vi "test_MonoGetConfig.vi"(6 "Delay between send and receive [ms]":i32=100, 7 "Test should pass":bool=TRUE, 8 "error in":errorcluster, 9 "tear down connection":bool=TRUE, 10 "set-up a connection":bool=TRUE, 11 "device selection":enum16{"monochromator", "CCD", "SCD"}(ring)) -> (0 "error out":errorcluster)   [LabVIEW 2023]
uses:
  Classes/Mono/configuration.ctl
  Classes/Mono/filterWheel.ctl
  Classes/Mono/grating.ctl
  Classes/Mono/mirror.ctl
  Classes/Mono/port.ctl
  Classes/Mono/Monochromator.lvclass
  C:/Projects/Horiba/horiba-labview-sdk/Source/Classes/GenericDevice/GenericDevice.lvclass
  <vilib>/addons/_JKI Toolkits/Caraya/classes/Assert/Assert Equal Value_Variant.vi
  <vilib>/addons/_JKI Toolkits/Caraya/classes/Assert/Assert Not Error.vi
  <vilib>/addons/_JKI Toolkits/Caraya/classes/Test/Test.lvclass
  <vilib>/addons/_JKI Toolkits/Caraya/classes/Assert/Assert.lvclass
  <vilib>/Hampel Software Engineering/HSE Logger/hse-logger.lvlib
panel:
  out "log-file path":path
  out "config-text pairs":string[][](array[string])=[["$.configuration.filterWheels", ""], ["$.configuration.gratings", "- blaze: 0\r  grooveDensity: 1800\r  positionIndex: 0\n- blaze: 0\r  grooveDensity: 1200\r  positionIndex: 1\n- blaze: 0\r  grooveDensity: 300\r  positionIndex: 2"], ["$.configuration.mirrors", "- location: 1\n- location: 2"], ["$.configuration.monoModel", "iHR320"], ["$.configuration.ports", "- monoPortLocation: 1\r  slitType: 2\n- monoPortLocation: 2\r  slitType: 2\n- monoPortLocation: 4\r  slitType: 2"], ["$.configuration.procuctId", "257"], ["$.configuration.serialNumber", ""]]
  out "config-JSON pairs":string[][](array[string])=[["$.configuration.filterWheels", "[]"], ["$.configuration.gratings", "[{\"blaze\":0,\"grooveDensity\":1800,\"positionIndex\":0},{\"blaze\":0,\"grooveDensity\":1200,\"positionIndex\":1},{\"blaze\":0,\"grooveDensity\":300,\"positionIndex\":2}]"], ["$.configuration.mirrors", "[{\"location\":1},{\"location\":2}]"], ["$.configuration.monoModel", "\"iHR320\""], ["$.configuration.ports", "[{\"monoPortLocation\":1,\"slitType\":2},{\"monoPortLocation\":2,\"slitType\":2},{\"monoPortLocation\":4,\"slitType\":2}]"], ["$.configuration.procuctId", "\"257\""], ["$.configuration.serialNumber", "\"\""]]
  out "config-JSON string":string="{\"configuration\":{\"CenterWavelength\":0,\"ChipHSpacing\":\"260\",\"ChipHeight\":\"256\",\"ChipName\":\"CCD30-11-1-275\",\"ChipSerialNumber\":\"20091-22-21\",\"ChipVSpacing\":\"260\",\"ChipWidth\":\"1024\",\"DeviceType\":\"HORIBA Scientific Syncerity\",\"FitParameters\":[0,1,0,0,0],\"Gains\":[{\"Info\":\"Best Dynamic Range\",\"Token\":1},{\"Info\":\"High Light\",\"Token\":0},{\"Info\":\"High Sensitivity\",\"Token\":2}],\"HardwareAvgAvailable\":\"False\",\"LineScan\":\"False\",\"ProductId\":\"13\",\"SerialNumber\":\"Camera SN:  2244\",\"Signals\":[{\"Events\":[{\"Name\":\"Ready For Trigger\",\"Token\":1,\"Types\":[{\"Name\":\"TTL Active Low\",\"Token\":1},{\"Name\":\"TTL Active High\",\"Token\":0}]},{\"Name\":\"Shutter Open\",\"Token\":3,\"Types\":[{\"Name\":\"TTL Active Low\",\"Token\":1},{\"Name\":\"TTL Active High\",\"Token\":0}]},{\"Name\":\"Start Experiment\",\"Token\":0,\"Types\":[{\"Name\":\"TTL Active Low\",\"Token\":1},{\"Name\":\"TTL Active High\",\"Token\":0}]},{\"Name\":\"Reserved-DO NOT USE\",\"Token\":2,\"Types\":[{\"Name\":\"TTL Active Low\",\"Token\":1},{\"Name\":\"TTL Active High\",\"Token\":0}]}],\"Name\":\"Signal Output\",\"Token\":0}],\"Speeds\":[{\"Info\":\" 1 MHz       \",\"Token\":1},{\"Info\":\"45 kHz       \",\"Token\":0},{\"Info\":\"500 kHz Wrap\",\"Token\":127},{\"Info\":\" 1 MHz Ultra \",\"Token\":2}],\"SupportedFeatures\":{\"CF_3PositionSlit\":\"False\",\"CF_CMOSOffsetCorrection\":\"False\",\"CF_Cleaning\":\"True\",\"CF_DSP\":\"False\",\"CF_DSPBin2X\":\"False\",\"CF_DelayAfterTrigger\":\"False\",\"CF_Delays\":\"False\",\"CF_EMCCD\":\"False\",\"CF_EShutter\":\"False\",\"CF_HDR\":\"False\",\"CF_Image\":\"True\",\"CF_MemorySlots\":\"True\",\"CF_Metadata\":\"False\",\"CF_MultipleExposeTimes\":\"False\",\"CF_MultipleSensors\":\"False\",\"CF_PulseSummation\":\"False\",\"CF_ROIs\":\"True\",\"CF_Signals\":\"True\",\"CF_Spectra\":\"True\",\"CF_TriggerQualifier\":\"False\",\"CF_Triggers\":\"True\"},\"Triggers\":[{\"Events\":[{\"Name\":\"Each - For Each Acq\",\"Token\":1,\"Types\":[{\"Name\":\"TTL Rising  Edge\",\"Token\":1},{\"Name\":\"TTL Falling Edge\",\"Token\":0}]},{\"Name\":\"Once - Start All\",\"Token\":0,\"Types\":[{\"Name\":\"TTL Rising  Edge\",\"Token\":1},{\"Name\":\"TTL Falling Edge\",\"Token\":0}]}],\"Name\":\"Trigger Input\",\"Token\":0}],\"Version\":\"Syncerity Ver 1.001.7.1\"}}"
  # "Connector Pane"
  # "Locals"
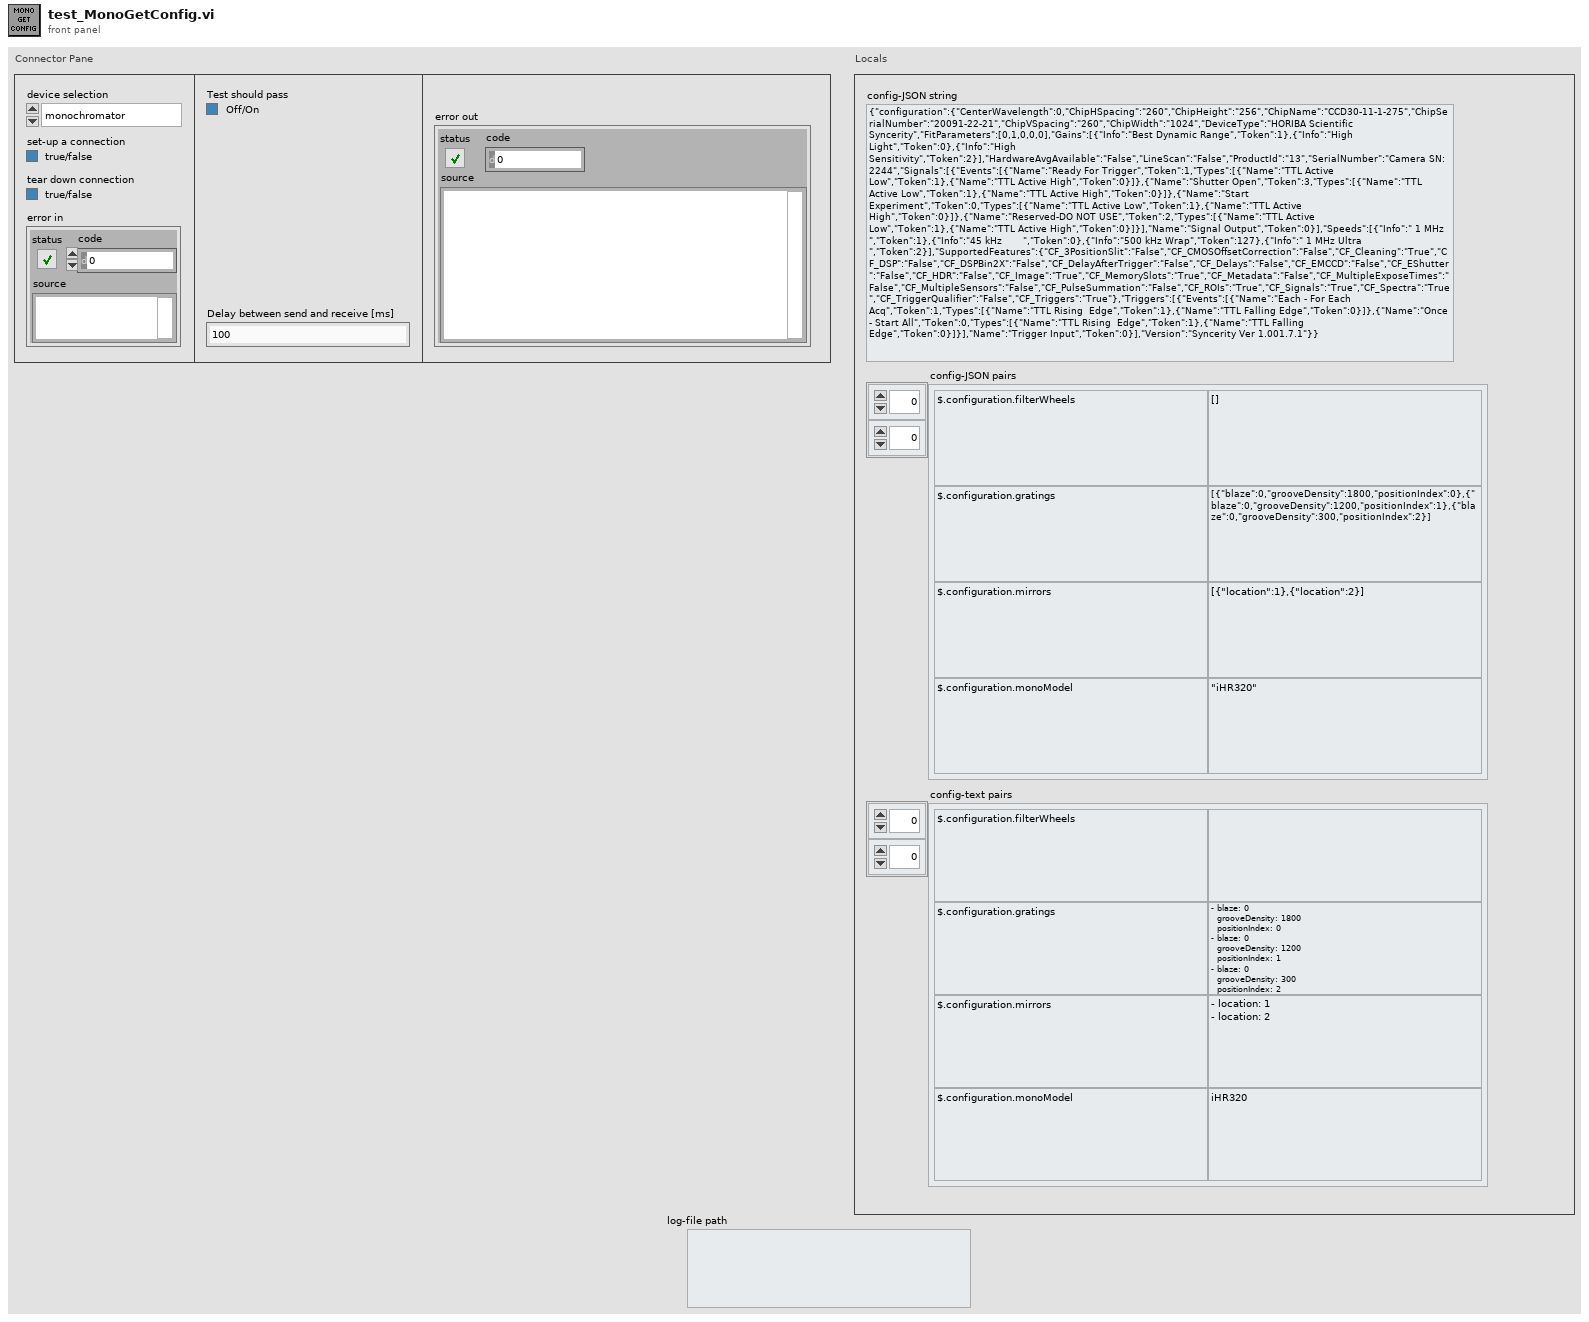
[diagram p1: front panel]
types:
  T1 = typedef "Monochromator.lvclass/configuration.ctl" = cluster{"filterWheels":T2[], "gratings":T3[], "mirrors":T4[], "model":string, "ports":T5[], "productId":string, "serialNumber":string}
  T2 = typedef "Monochromator.lvclass/filterWheel.ctl" = cluster{"locationId":i32}
  T3 = typedef "Monochromator.lvclass/grating.ctl" = cluster{"blaze":i32, "grooveDensity":i32, "positionIndex":i32}
  T4 = typedef "Monochromator.lvclass/mirror.ctl" = cluster{"locationId":i32}
  T5 = typedef "Monochromator.lvclass/port.ctl" = cluster{"locationId":i32, "slitType":i32}
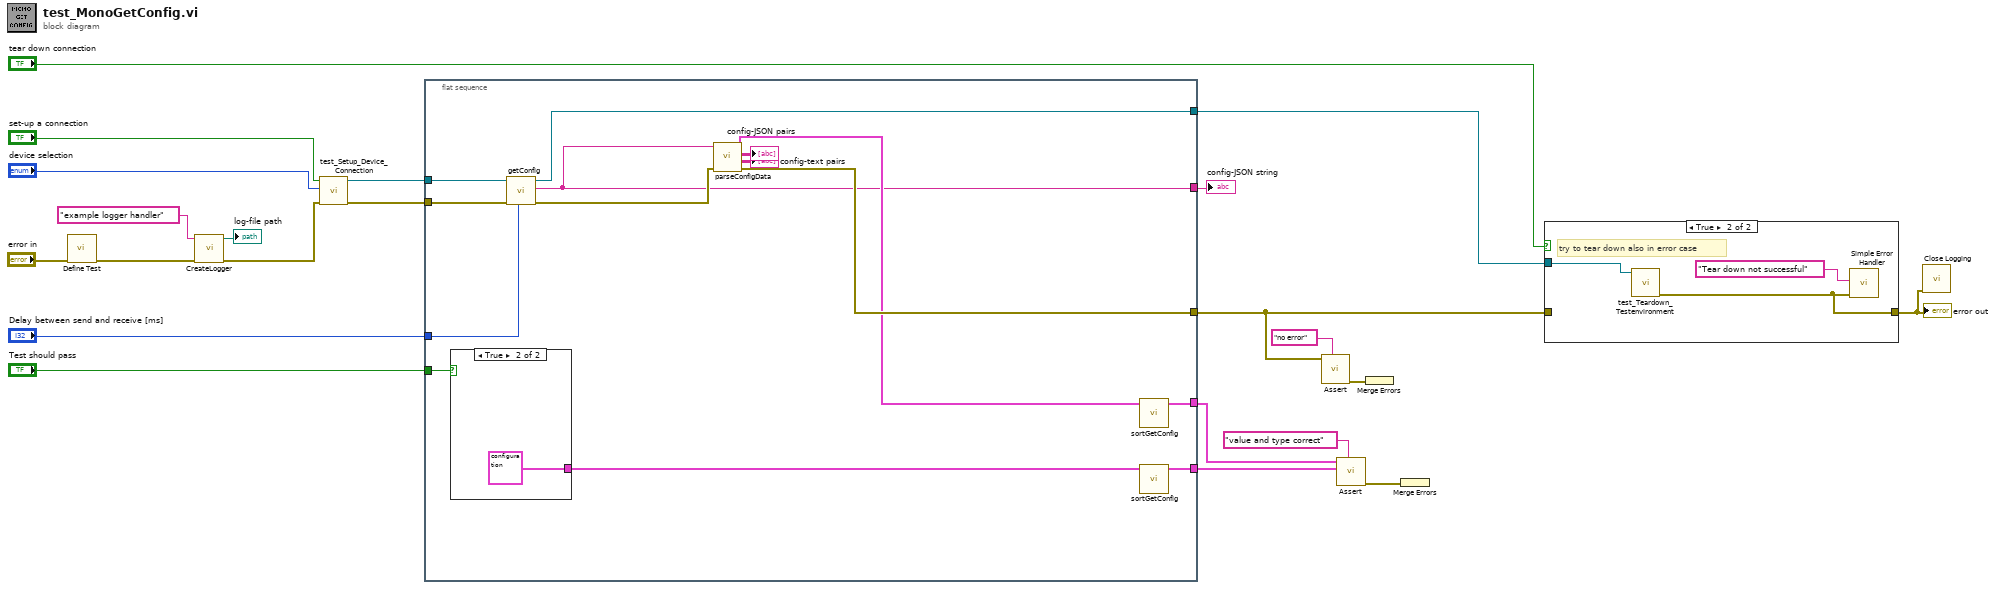
[diagram p0: block diagram]
diagram:
  n1 = call <vilib>:"Define Test.vi"("error in (no error)"="error in") -> ("error out"=w3:errorcluster)  [unwired: 9 in, 1 out]
  n2 = call "CreateLogger.vi"("error in (no error)"=w3, "Handler Name"="example logger handler") -> ("error out"=w2:errorcluster, "log-file path"=→"log-file path":path)  [unwired: 8 in]
  n3 = call "test_Setup_Device_Connection.vi"("error in (no error)"=w2, "device selection"="device selection", "set-up a connection"="set-up a connection") -> ("error out"=w10:errorcluster, "Monochromator.lvclass"=w7:refnum<class "Monochromator.lvclass">)  [unwired: 5 in, 2 out]
  n4 = flat-sequence {
    tunnel: [w26] -> w20
    tunnel: w10 -> [w36]
    tunnel: w7 -> [w35]
    tunnel: [w30] -> w14
    tunnel: "Test should pass" -> [w34]
    tunnel: [w33] -> w13
    tunnel: "Delay between send and receive [ms]" -> [w32]
    tunnel: [w23] -> w8
    tunnel: [w25] -> w6
    frame #0 {
      n5 = case shown="True" w34 {
        tunnel: [_ T1 {"filterWheels"=[], "gratings"=[{"blaze"=0, "grooveDensity"=1800, "positionIndex"=0}, {"blaze"=0, "grooveDensity"=1200, "positionIndex"=1}, {"blaze"=0, "grooveDensity"=300, "positionIndex"=2}], "mirrors"=[{"locationId"=1}, {"locationId"=2}], "model"="iHR320", "ports"=[{"locationId"=1, "slitType"=1}, {"locationId"=2, "slitType"=1}, {"locationId"=4, "slitType"=1}], "productId"="257", "serialNumber"=""} ("unsorted 2")] -> w24
        frame False {
        }
        frame True {
        }
      }
      n6 = call "getConfig.vi"("Delay between send and receive [ms]"=w32, "error in (no error)"=w36, "Monochromator in"=w35) -> ("error out"=w31:errorcluster, "config-JSON string"=w26:string, "Monochromator out"=w33:refnum<class "Monochromator.lvclass">)  [unwired: 6 in]
      n7 = call "parseConfigData.vi"("error in (no error)"=w31, "results-JSON string"=w26) -> ("error out"=w30:errorcluster, "config-text pairs"=→"config-text pairs":string[][], "config-JSON pairs"=→"config-JSON pairs":string[][], "config data"=w27:T1)  [unwired: 6 in]
      n8 = call "sortGetConfig.vi"("config data in"=w27) -> ("config data out"=w25:T1)  [unwired: 10 in]
      n9 = call "sortGetConfig.vi"("config data in"=w24) -> ("config data out"=w23:T1)  [unwired: 10 in]
    }
  }
  n10 = call-poly <vilib>:"Assert.vi"("Label"="no error" ("Label (VI Title)"), "Not Error?"=w14) -> ("error out"=w16:errorcluster)  [unwired: 8 in, 1 out]
  n11 = call-poly <vilib>:"Assert.vi"("Label"="value and type correct" ("Label (VI Title)"), "Y"=w8, "X"=w6) -> ("error out"=w21:errorcluster)  [unwired: 7 in, 1 out]
  n12 = Merge Errors(w16) -> ()  [unwired: 1 out]
  n13 = Merge Errors(w21) -> ()  [unwired: 1 out]
  n14 = case shown="True" "tear down connection" {
    tunnel: w13 -> [_ w40]
    tunnel: [w38 w39] -> w1
    tunnel: w14 -> [w38 _]
    frame False {
    }
    frame True {
      # "try to tear down also in error case"
      n15 = call "test_Teardown_Testenvironment.vi"("GenericDevice.lvclass"=w40) -> ("error out"=w39:errorcluster)  [unwired: 9 in, 1 out]
      n16 = call <vilib>:"Simple Error Handler.vi"("error source (\" \")"="Tear down not successful" ("error source (\" \")"), "error in (no error)"=w39) -> ()  [unwired: 3 in, 5 out]
    }
  }
  "error out" <- w1
  n17 = call <vilib>:"Close Logging.vi"("error in"=w1) -> ()  [unwired: 10 in, 1 out]
  "config-JSON string" <- w20
